vi "convertDCIMGsInFileToTifStack.vi"(1 "fileExtension":string="dcimg", 2 "path":path=path "C:/Users/sims01/Desktop/dataTest_v1") -> (0 "stackConvComplete":bool)   [LabVIEW 2015]
panel:
  out "appended path":path
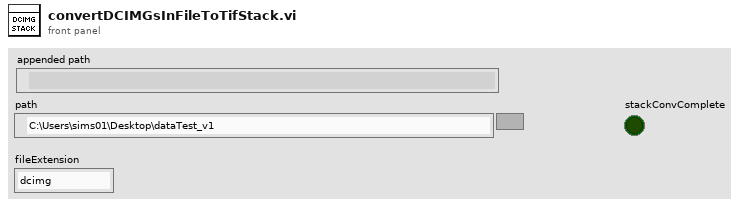
[diagram p1: front panel]
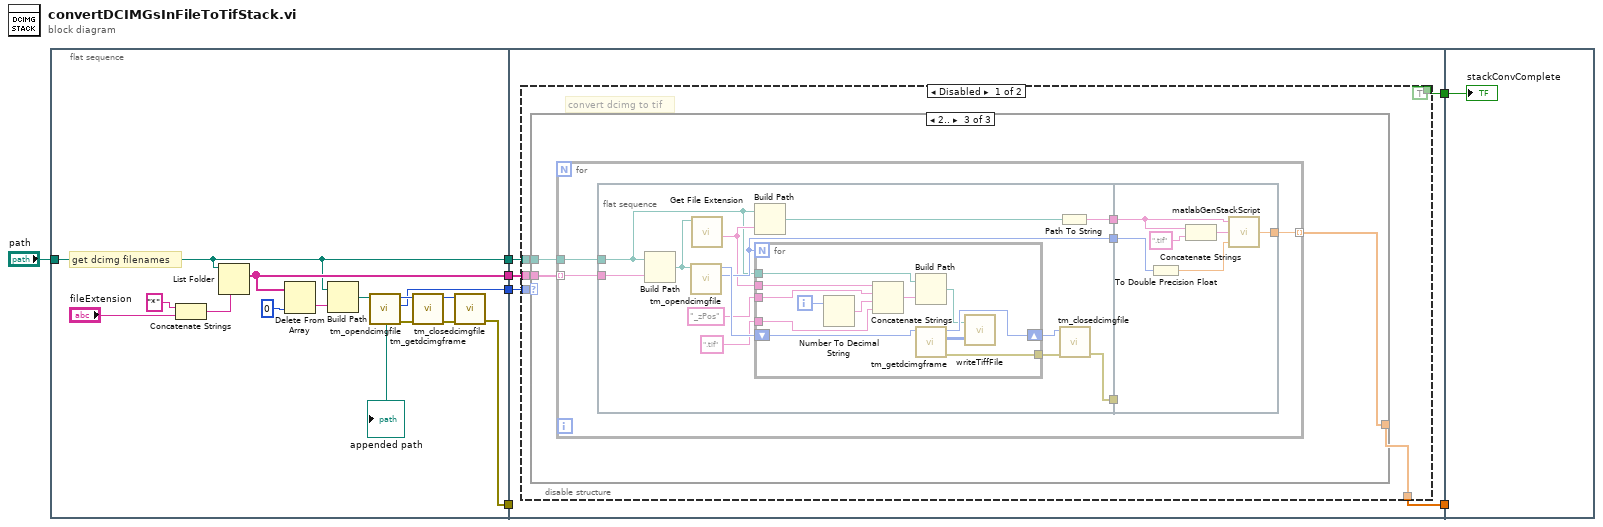
[diagram p0: block diagram]
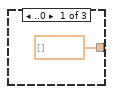
[diagram p2: hidden frame]
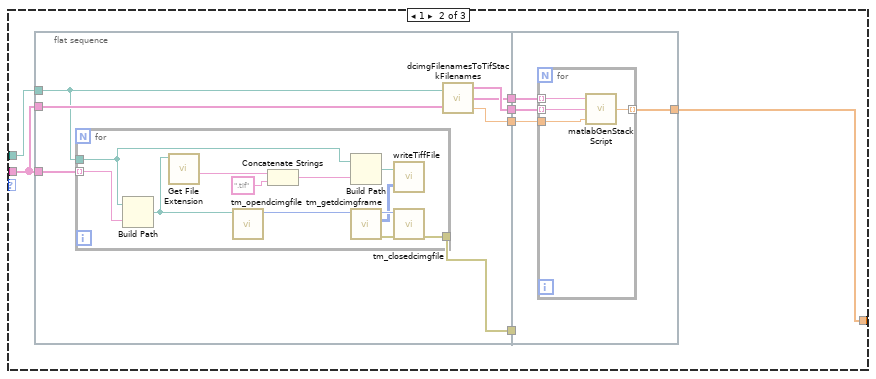
[diagram p3: hidden frame]
diagram:
  n1 = flat-sequence {
    tunnel: [w12] -> w7
    tunnel: "path" -> [w9]
    tunnel: [w11] -> w5
    tunnel: [w9] -> w4
    tunnel: [w10] -> w3
    tunnel: w7 -> [_]
    tunnel: w5 -> [w24]
    tunnel: w4 -> [w25]
    tunnel: w3 -> [w26]
    tunnel: [w23] -> w2
    tunnel: [w22] -> w1
    tunnel: w2 -> [_]
    tunnel: w1 -> [w107]
    frame #0 {
      # "get dcimg filenames"
      n2 = Concatenate Strings("*" ("string"), "fileExtension") -> (w20:string)
      n3 = List Folder(path=w9, pattern=w20) -> (filenames=w11:string[])  [unwired: 2 in, 3 out]
      n4 = Delete From Array(array=w11, index=0) -> (deleted portion=w18:string)  [unwired: 1 in, 1 out]
      n5 = Build Path(base path=w9, name or relative path=w18) -> (appended path=w17:path)
      "appended path" <- w17
      n6 = call <userlib>:"tm_opendcimgfile.vi"("Path"=w17) -> ("error out"=w15:errorcluster, "Total Frames"=w10:i32, "File Handle"=w16:u32)  [unwired: 8 in]
      n7 = call <userlib>:"tm_getdcimgframe.vi"("error in (no error)"=w15, "File Handle in"=w16) -> ("error out"=w13:errorcluster, "File Handle out"=w14:u32)  [unwired: 6 in, 2 out]
      n8 = call <userlib>:"tm_closedcimgfile.vi"("error in (no error)"=w13, "File Handle"=w14) -> ("error out"=w12:errorcluster)  [unwired: 9 in]
    }
    frame #1 {
      n9 = disable-structure shown="Disabled" {
        disable-tunnel: w26 -> [w31 _]
        disable-tunnel: w25 -> [w30 _]
        disable-tunnel: w24 -> [w29 _]
        disable-tunnel: [w28 _] -> w23
        disable-tunnel: [TRUE _] -> w22
        frame Disabled {
          # "convert dcimg to tif"
          n10 = case shown="2.." w31 {
            tunnel: w30 -> [_ w39 w69]
            tunnel: w29 -> [_ w38 w68]
            tunnel: [dbl[] [] w33 w67] -> w28
            frame ..0 {
            }
            frame 1 {
              n11 = flat-sequence {
                tunnel: w39 -> [w40]
                tunnel: w38 -> [w46]
                tunnel: w38 -> [w41]
                tunnel: [w45] -> w37
                tunnel: [w44] -> w36
                tunnel: [w43] -> w35
                tunnel: [w42] -> w34
                tunnel: w37 -> [_]
                tunnel: w36 -> [w62]
                tunnel: w35 -> [w61]
                tunnel: w34 -> [w60]
                tunnel: [w59] -> w33
                frame #0 {
                  n12 = for {
                    tunnel: w46 -> [w58] mode=indexing
                    tunnel: w40 -> [w54]
                    tunnel: [w47] -> w45
                    n13 = Build Path(base path=w54, name or relative path=w58) -> (appended path=w57:path)
                    n14 = call <vilib>:"Get File Extension.vi"("file"=w57) -> ("filename without extension"=w56:string)  [unwired: 6 in, 4 out]
                    n15 = call <userlib>:"tm_opendcimgfile.vi"("Path"=w57) -> ("File Handle"=w53:u32)  [unwired: 8 in, 2 out]
                    n16 = Concatenate Strings(w56, ".tif" ("string")) -> (w52:string)
                    n17 = Build Path(base path=w54, name or relative path=w52) -> (appended path=w48:path)
                    n18 = call <userlib>:"tm_getdcimgframe.vi"("File Handle in"=w53) -> ("error out"=w51:errorcluster, "Data"=w49:u16[][], "File Handle out"=w50:u32)  [unwired: 7 in, 1 out]
                    n19 = call "writeTiffFile.vi"("Image Pixels (U16)"=w49, "File Path"=w48) -> ()
                    n20 = call <userlib>:"tm_closedcimgfile.vi"("error in (no error)"=w51, "File Handle"=w50) -> ("error out"=w47:errorcluster)  [unwired: 9 in]
                  }
                  n21 = call "dcimgFilenamesToTifStackFilenames.vi"("Base path"=w40, "filenames"=w41) -> ("tifStackFnames"=w44:string[], "stackFnames"=w43:string[], "noImgsInStack"=w42:dbl)
                }
                frame #1 {
                  n22 = for {
                    tunnel: w62 -> [w65] mode=indexing
                    tunnel: w61 -> [w66] mode=indexing
                    tunnel: w60 -> [w64]
                    tunnel: [w63] -> w59 mode=indexing
                    n23 = call "matlabGenStackScript.vi"("noImgsInStack"=w64, "tifStackFname"=w65, "stackFnameBase"=w66) -> ("No stacksGenerated"=w63:dbl)
                  }
                }
              }
            }
            frame 2.. {
              n24 = for {
                tunnel: w68 -> [w75] mode=indexing
                tunnel: w69 -> [w74]
                tunnel: [w70] -> w67 mode=indexing
                n25 = flat-sequence {
                  tunnel: w75 -> [w88]
                  tunnel: w74 -> [w78]
                  tunnel: [w83] -> w73
                  tunnel: [w76] -> w72
                  tunnel: [w80] -> w71
                  tunnel: w73 -> [_]
                  tunnel: w72 -> [w105]
                  tunnel: w71 -> [w103]
                  tunnel: [w101] -> w70
                  frame #0 {
                    n26 = Build Path(base path=w78, name or relative path=w88) -> (appended path=w87:path)
                    n27 = call <userlib>:"tm_opendcimgfile.vi"("Path"=w87) -> ("Total Frames"=w80:i32, "File Handle"=w86:u32)  [unwired: 8 in, 1 out]
                    n28 = call <vilib>:"Get File Extension.vi"("file"=w87) -> ("filename without extension"=w79:string)  [unwired: 6 in, 4 out]
                    n29 = Build Path(base path=w78, name or relative path=w79) -> (appended path=w77:path)
                    n30 = for {
                      N: w80 -> [_]
                      tunnel: [w99] -> w85
                      shift-right: [w98] -> w84
                      shift-left: w86 -> [w100]
                      tunnel: w78 -> [w95]
                      tunnel: "_zPos" -> [w92]
                      tunnel: w79 -> [w91]
                      tunnel: ".tif" ("string") -> [w89]
                      i -> [w96]
                      n31 = Number To Decimal String(number=w96) -> (decimal integer string=w90:string)  [unwired: 1 in]
                      n32 = Concatenate Strings(w91, w92, w90, w89) -> (w94:string)
                      n33 = Build Path(base path=w95, name or relative path=w94) -> (appended path=w93:path)
                      n34 = call <userlib>:"tm_getdcimgframe.vi"("File Handle in"=w100) -> ("error out"=w99:errorcluster, "Data"=w97:u16[][], "File Handle out"=w98:u32)  [unwired: 7 in, 1 out]
                      n35 = call "writeTiffFile.vi"("Image Pixels (U16)"=w97, "File Path"=w93) -> ()
                    }
                    n36 = Path To String(path=w77) -> (string=w76:string)
                    n37 = call <userlib>:"tm_closedcimgfile.vi"("error in (no error)"=w85, "File Handle"=w84) -> ("error out"=w83:errorcluster)  [unwired: 9 in]
                  }
                  frame #1 {
                    n38 = To Double Precision Float(number=w103) -> (double precision float=w102:dbl)
                    n39 = Concatenate Strings(w105, ".tif" ("string")) -> (w104:string)
                    n40 = call "matlabGenStackScript.vi"("noImgsInStack"=w102, "tifStackFname"=w104, "stackFnameBase"=w105) -> ("No stacksGenerated"=w101:dbl)
                  }
                }
              }
            }
          }
        }
        frame Enabled {
        }
      }
    }
    frame #2 {
      "stackConvComplete" <- w107
    }
  }
